vi "Command Handler.vi"   [LabVIEW 2020]
uses:
  Type Definitions/Data Frame.ctl
  Type Definitions/Data Frame Header.ctl
  Type Definitions/Payload Class.ctl
  Type Definitions/Device.ctl
  Type Definitions/Enum - Data.ctl
  Type Definitions/Notification Data.ctl
  Type Definitions/Enum - Notification Types.ctl
  Type Definitions/Analog Output Command.ctl
  Type Definitions/Digital Output Command.ctl
types:
  T1 = typedef "Enum - Data.ctl" = enum16{"Analog Input Data", "Notification Data", "Analog Output Data", "Digital Output Data", "Command Ack", "Digital Input Data", "GPS Solution Data"}
  T2 = typedef "Payload Class.ctl" = enum16{"System State", "Parameters", "Metadata", "Software Monitor", "Data", "Commands"}
  T3 = typedef "Data Frame.ctl" = cluster{"Frame Header":T4, "Payload":string, "CRC":u32}
  T4 = typedef "Data Frame Header.ctl" = cluster{"Sync":u32, "Time":dbl, "Nanosecond Counter":i64, "Payload Class":T2, "Payload ID":u16, "Counter":i32, "Options":u32, "Source":T5, "Destination":T5}
  T5 = typedef "Device.ctl" = enum32{"None", "Exec", "Aux1", "Aux2", "Aux3"}
  T6 = typedef "Enum - Notification Types.ctl" = enum16{"Warning", "Acknowledge", "Notification"}
  T7 = typedef "Notification Data.ctl" = cluster{"Notification Type":T6, "Code":i32, "Description":string}
  T8 = typedef "Analog Output Command.ctl" = cluster{"AO Channel":u8, "State":dbl}
  T9 = typedef "Digital Output Command.ctl" = cluster{"DO Channel":u8, "State":bool}
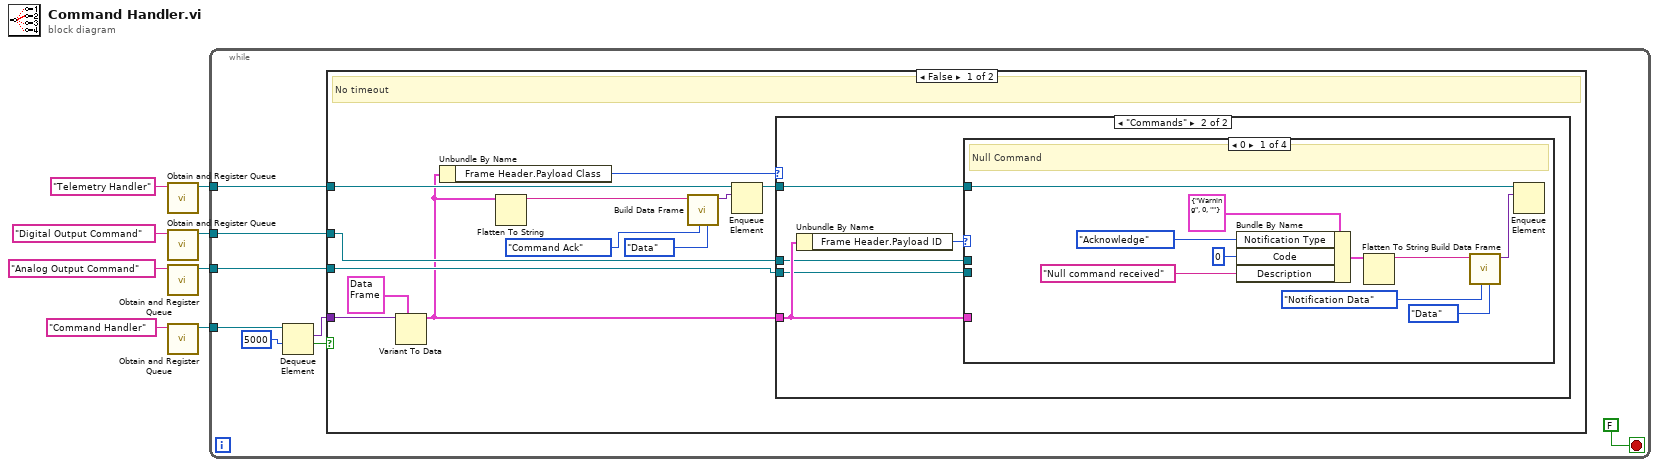
[diagram p0: block diagram]
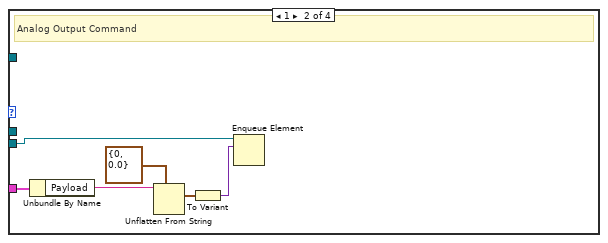
[diagram p3: hidden frame]
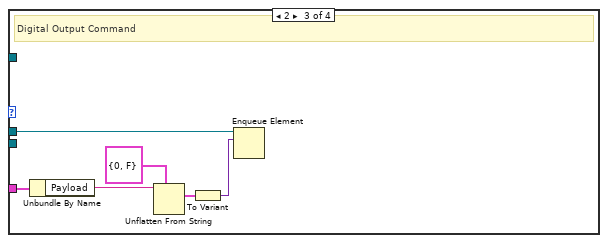
[diagram p4: hidden frame]
diagram:
  n1 = call "Obtain and Register Queue.vi"("name (unnamed)"="Telemetry Handler") -> ("Queue Out"=w6:refnum<queue>)  [unwired: 7 in, 3 out]
  n2 = call "Obtain and Register Queue.vi"("name (unnamed)"="Digital Output Command") -> ("Queue Out"=w3:refnum<queue>)  [unwired: 7 in, 3 out]
  n3 = call "Obtain and Register Queue.vi"("name (unnamed)"="Analog Output Command") -> ("Queue Out"=w1:refnum<queue>)  [unwired: 7 in, 3 out]
  n4 = call "Obtain and Register Queue.vi"("name (unnamed)"="Command Handler") -> ("Queue Out"=w5:refnum<queue>)  [unwired: 7 in, 3 out]
  n5 = while {
    tunnel: w6 -> [w15]
    tunnel: w5 -> [w12]
    tunnel: w1 -> [w14]
    tunnel: w3 -> [w13]
    stop <- FALSE stop-if-true
    n6 = Dequeue Element(queue=w12, timeout in ms (-1)=5000) -> (element=w11:variant, timed out?=w9:bool)  [unwired: 1 in, 2 out]
    n7 = case shown="False" w9 {
      tunnel: w15 -> [w28 _]
      tunnel: w14 -> [w27 _]
      tunnel: w13 -> [w26 _]
      tunnel: w11 -> [w17 _]
      frame False {
        # "No timeout"
        n8 = Variant To Data(type=T3 {"Frame Header"={"Sync"=0, "Time"=0.0, "Nanosecond Counter"=0, "Payload Class"=enum."System State", "Payload ID"=0, "Counter"=0, "Options"=0, "Source"=enum."None", "Destination"=enum."None"}, "Payload"="", "CRC"=0} ("Frame"), Variant=w17) -> (data=w22:T3)  [unwired: 1 in, 1 out]
        n9 = Unbundle By Name(w22) -> ("Frame Header.Payload Class"=w24:T2)
        n10 = Flatten To String(anything=w22) -> (data string=w21:string)  [unwired: 3 in, 2 out]
        n11 = call "Build Data Frame.vi"("Payload Class (Data)"=Payload_Class."Data", "Payload ID (0)"=Enum_-_Data."Command Ack" ("Data"), "Payload (Empty String)"=w21) -> ("Frame"=w18:variant)  [unwired: 7 in, 1 out]
        n12 = Enqueue Element(queue=w28, element=w18) -> (queue out=w23:refnum<queue>)  [unwired: 2 in, 2 out]
        n13 = case shown="\"Commands\"" w24 {
          tunnel: w22 -> [_ w32]
          tunnel: w23 -> [_ w31]
          tunnel: w27 -> [_ w30]
          tunnel: w26 -> [_ w29]
          frame Default {
          }
          frame "Commands" {
            n14 = Unbundle By Name(w32) -> ("Frame Header.Payload ID"=w33:u16)
            n15 = case shown="0" w33 {
              tunnel: w32 -> [_ w49 w55 _]
              tunnel: w31 -> [w43 _ _ _]
              tunnel: w30 -> [_ w45 _ _]
              tunnel: w29 -> [_ _ w52 _]
              frame 0 {
                # "Null Command"
                n16 = Bundle By Name(cluster=T7 {"Notification Type"=enum."Warning", "Code"=0, "Description"=""}, "Notification Type"=Enum_-_Notification_Types."Acknowledge", "Code"=0, "Description"="Null command received") -> (w35:T7)
                n17 = Flatten To String(anything=w35) -> (data string=w40:string)  [unwired: 3 in, 2 out]
                n18 = call "Build Data Frame.vi"("Payload Class (Data)"=Payload_Class."Data", "Payload ID (0)"=Enum_-_Data."Notification Data" ("Data"), "Payload (Empty String)"=w40) -> ("Frame"=w42:variant)  [unwired: 7 in, 1 out]
                n19 = Enqueue Element(queue=w43, element=w42) -> ()  [unwired: 2 in, 3 out]
              }
              frame 1 {
                # "Analog Output Command"
                n20 = Unbundle By Name(w49) -> ("Payload"=w48:string)
                n21 = Unflatten From String(type=T8 {"AO Channel"=0, "State"=0.0} ("Analog Output Command"), binary string=w48) -> (value=w46:T8)  [unwired: 3 in, 2 out]
                n22 = To Variant(anything=w46) -> (Variant=w44:variant)
                n23 = Enqueue Element(queue=w45, element=w44) -> ()  [unwired: 2 in, 3 out]
              }
              frame 2 {
                # "Digital Output Command"
                n24 = Unbundle By Name(w55) -> ("Payload"=w54:string)
                n25 = Unflatten From String(type=T9 {"DO Channel"=0, "State"=FALSE}, binary string=w54) -> (value=w51:T9)  [unwired: 3 in, 2 out]
                n26 = To Variant(anything=w51) -> (Variant=w50:variant)
                n27 = Enqueue Element(queue=w52, element=w50) -> ()  [unwired: 2 in, 3 out]
              }
              frame Default {
                # "Unhandled Command"
              }
            }
          }
        }
      }
      frame True {
        # "Timed out"
      }
    }
  }
